vi "Bernoulli PF.vi"(9 "p":dbl=0.2, 11 "x":i32) -> (0 "error":i32, 3 "prob(x)":dbl=0.8)   [LabVIEW 2017, in "NI_Gmath.lvlib"]
doc: "Computes the discrete probability function (PF), or the probability that the random variate X, where X describes the selected distribution type, takes on the value <B>n</B>. You must manually select the polymorphic instance to use."
uses:
  NI_Gmath.lvlib
  st_error_code.ctl
panel:
  # "Bernoulli PF"
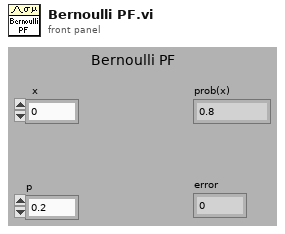
[diagram p1: front panel]
types:
  T1 = typedef "NI_Gmath.lvlib/st_error_code.ctl" = i32
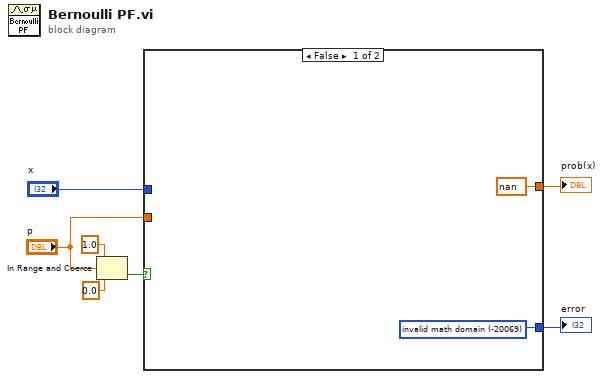
[diagram p0: block diagram]
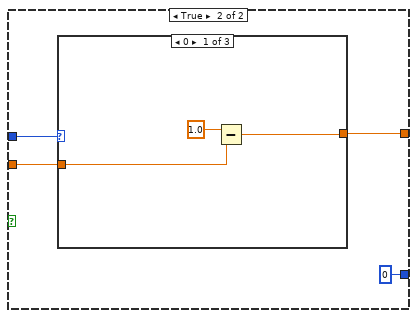
[diagram p2: hidden frame]
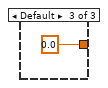
[diagram p4: hidden frame]
diagram:
  n1 = In Range and Coerce(upper limit=1.0, x="p", lower limit=0.0) -> (In Range?=w5:bool)  [unwired: 1 out]
  n2 = case shown="False" w5 {
    tunnel: [w8 0 ("invalid math domain")] -> w1
    tunnel: "p" -> [_ w10]
    tunnel: "x" -> [_ w12]
    tunnel: [nan w11] -> w2
    frame False {
      w8 = T1 -20069 items=["invalid math domain"=-20069, "Fourier interpolation size m >= n"=-20070, "empty array"=-20003] ("stat interp error code")
    }
    frame True {
      n3 = case shown="0" w12 {
        tunnel: [w14 w17 0.0 ("pdf(x)")] -> w11
        tunnel: w10 -> [w15 w17 _]
        frame 0 {
          n4 = Subtract(x=1.0, y=w15) -> (x-y=w14:dbl)
        }
        frame 1 {
        }
        frame Default {
        }
      }
    }
  }
  "prob(x)" <- w2
  "error" <- w1
